vi "DAQ Engine.vi"(8 "Error In":errorcluster, 10 "Output \nIndicator":T2=[FALSE, FALSE] caption="Z     Y     X", 11 "DAQ Action":T3) -> (0 "Error Out":errorcluster, 2 "Reset ?":bool, 3 "L       E \nIndicator":T1 caption="L      E")   [LabVIEW 2023]
doc: "VI for realizing DAQ action engine"
uses:
  <vilib>/DAQmx/create/channels.llb/DAQmx Create Channel (AI-Voltage-Basic).vi
  controls/Boolean L E indictaor.ctl
  controls/enum defining DAQ actions.ctl
  controls/Boolean output indicator.ctl
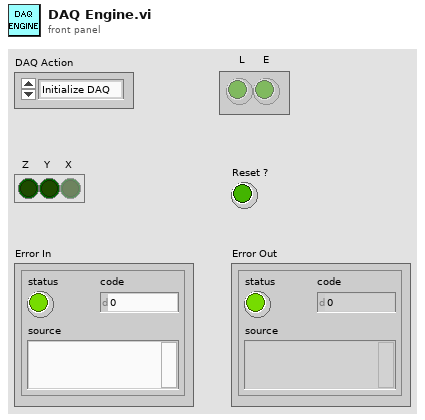
[diagram p1: front panel]
types:
  T1 = typedef "Boolean L E indictaor.ctl" = bool[]
  T2 = typedef "Boolean output indicator.ctl" = bool[]
  T3 = typedef "enum defining DAQ actions.ctl" = enum16{"Initialize DAQ", "Read L and  E  Commands", "Read R Command", "Write Outputs X, Y, and Z", "Release DAQ"}
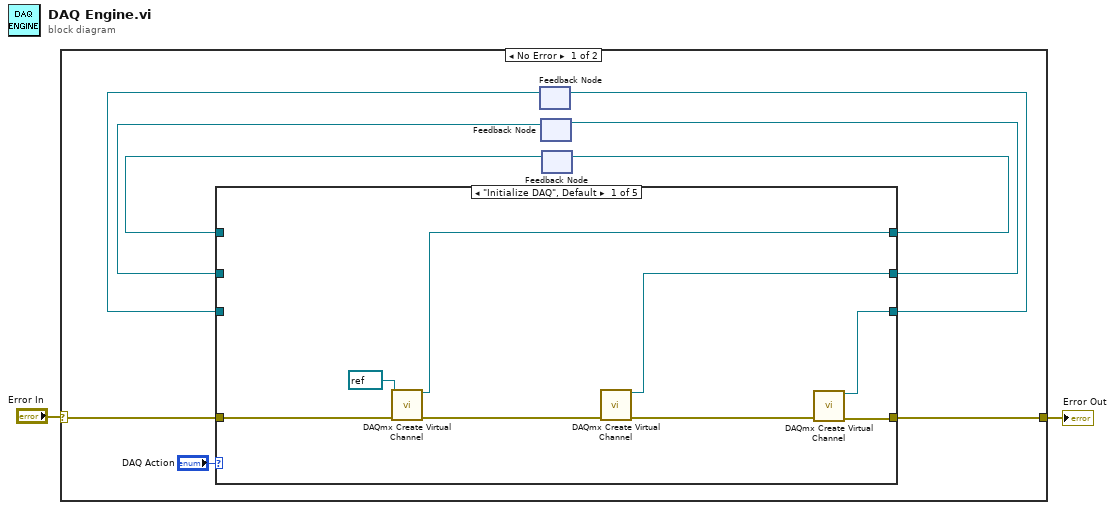
[diagram p0: block diagram]
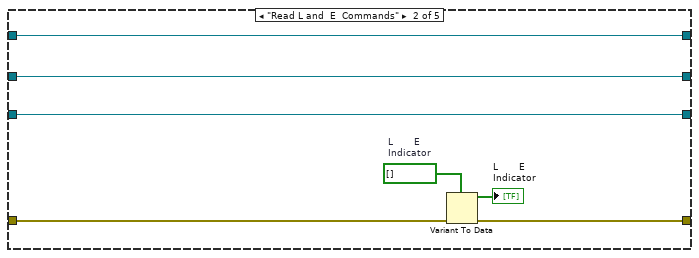
[diagram p2: hidden frame]
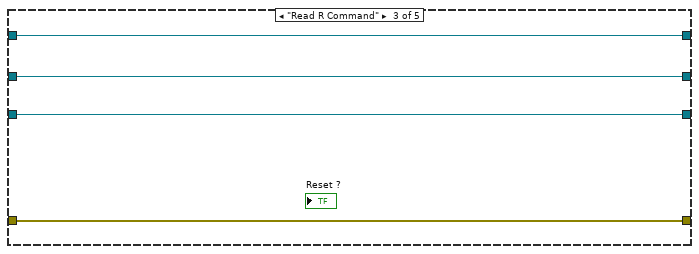
[diagram p3: hidden frame]
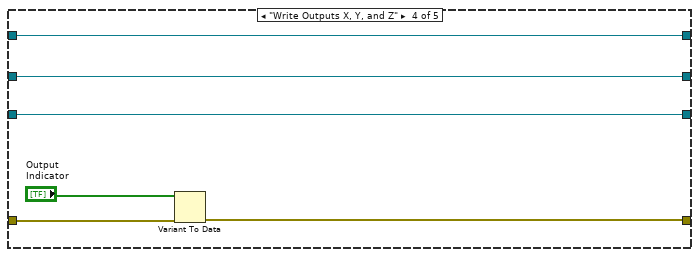
[diagram p4: hidden frame]
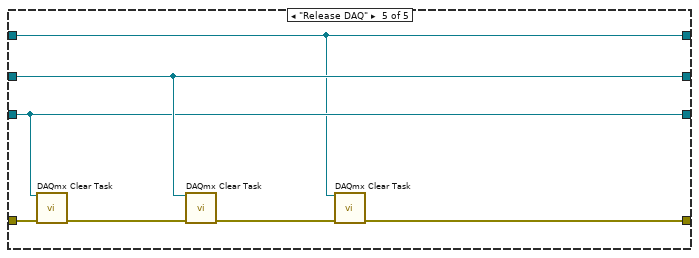
[diagram p5: hidden frame]
diagram:
  n1 = case shown="No Error" "Error In" {
    selector: "Error In" -> [w7 w44]
    tunnel: [w6 w44] -> w1
    frame No Error {
      n2 = feedback #1() -> (w4:refnum<k21>)  [unwired: 1 in]
      n3 = feedback #2() -> (w9:refnum<k21>)  [unwired: 1 in]
      n4 = feedback #3() -> (w8:refnum<k21>)  [unwired: 1 in]
      n5 = case shown="\"Initialize DAQ\", Default" "DAQ Action" {
        tunnel: [w18 w26 w27 w36 w41] -> w10
        tunnel: w9 -> [_ w26 w27 w36 w41]
        tunnel: w8 -> [_ w23 w28 w35 w37]
        tunnel: w7 -> [w17 w25 w30 w33 w40]
        tunnel: [w15 w22 w30 w34 w42] -> w6
        tunnel: [w14 w24 w29 w32 w38] -> w5
        tunnel: w4 -> [_ w24 w29 w32 w38]
        tunnel: [w13 w23 w28 w35 w37] -> w3
        frame "Initialize DAQ", Default {
          n6 = call-poly <vilib>:"DAQmx Create Virtual Channel.vi"("task in"=refnum<k21> refnum, "error in"=w17) -> ("task out"=w13:refnum<k21>, "error out"=w19:errorcluster)  [unwired: 12 in]
          n7 = call-poly <vilib>:"DAQmx Create Virtual Channel.vi"("error in"=w19) -> ("task out"=w18:refnum<k21>, "error out"=w16:errorcluster)  [unwired: 13 in]
          n8 = call-poly <vilib>:"DAQmx Create Virtual Channel.vi"("error in"=w16) -> ("task out"=w14:refnum<k21>, "error out"=w15:errorcluster)  [unwired: 13 in]
        }
        frame "Read L and  E  Commands" {
          w21 = T1 []  # L       E  Indicator
          n9 = Variant To Data(error in=w25, type=w21) -> (data=→"L       E \nIndicator":T1, error out=w22:errorcluster)  [unwired: 1 in]
        }
        frame "Read R Command" {
        }
        frame "Write Outputs X, Y, and Z" {
          n10 = Variant To Data(error in=w33, Variant="Output \nIndicator") -> (error out=w34:errorcluster)  [unwired: 1 in, 1 out]
        }
        frame "Release DAQ" {
          n11 = call <vilib>:"DAQmx Clear Task.vi"("task in"=w38, "error in"=w40) -> ("error out"=w39:errorcluster)  [unwired: 13 in]
          n12 = call <vilib>:"DAQmx Clear Task.vi"("task in"=w41, "error in"=w39) -> ("error out"=w43:errorcluster)  [unwired: 13 in]
          n13 = call <vilib>:"DAQmx Clear Task.vi"("task in"=w37, "error in"=w43) -> ("error out"=w42:errorcluster)  [unwired: 13 in]
        }
      }
      n14 = feedback-in #1(w5) -> ()
      n15 = feedback-in #2(w10) -> ()
      n16 = feedback-in #3(w3) -> ()
    }
    frame Error {
    }
  }
  "Error Out" <- w1
